vi "Cleanup.vi"(8 "error in (no error)":errorcluster, 11 "TermBuffer in":refnum<class "TermBuffer.lvclass">) -> (0 "error out":errorcluster)   [LabVIEW 2020, in "Terminal.lvlib" / "TermBuffer.lvclass"]
uses:
  TermBuffer.lvclass
  TermBuffer.lvclass/TermBuffer.ctl
  TermLine/TermLine.lvclass
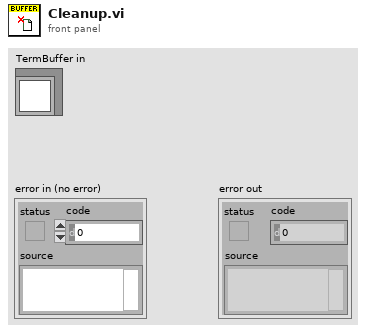
[diagram p1: front panel]
types:
  T1 = typedef "Terminal.lvlib/TermBuffer.lvclass/Ref Data.ctl" = cluster{"Lines":refnum<class "TermLine.lvclass">[], "Rows":i32, "Cols":i32}
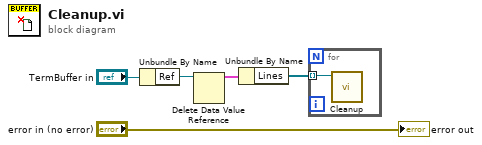
[diagram p0: block diagram]
diagram:
  n1 = Unbundle By Name("TermBuffer in") -> ("Ref"=w3:refnum<data-value>)
  n2 = Delete Data Value Reference(data value reference=w3) -> (data value=w2:T1)  [unwired: 1 in, 1 out]
  n3 = Unbundle By Name(w2) -> ("Lines"=w1:refnum<class "TermLine.lvclass">[])
  n4 = for {
    tunnel: w1 -> [w6] mode=indexing
    n5 = call "Cleanup.vi"("TermLine in"=w6) -> ()  [unwired: 10 in, 1 out]
  }
  "error out" <- "error in (no error)"
